vi "Non Linear Decimation on X by Min-Max Algorythm.vi"(6 "Width":u32, 8 "error in (no error)":errorcluster, 9 "Min Index":i32, 10 "Max Index":i32, 11 "Data To Decimate":dbl[](array[numeric])) -> (0 "error out":errorcluster, 3 "Decimated Data":dbl[](array[numeric]), 4 "Packet size":i32[](array[numeric]))   [LabVIEW 2022 SP3, in "Decimation.lvlib"]
uses:
  Decimation.lvlib
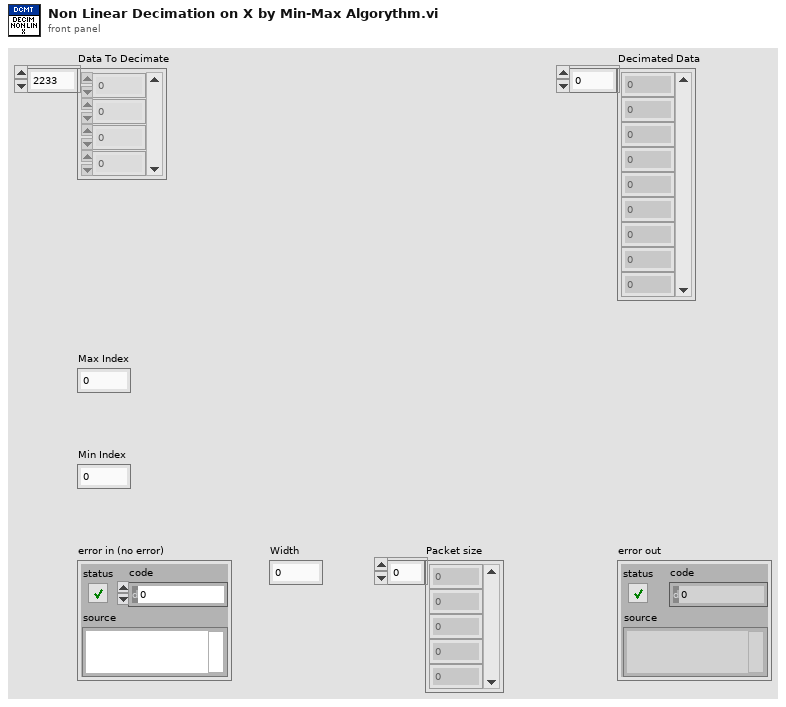
[diagram p1: front panel]
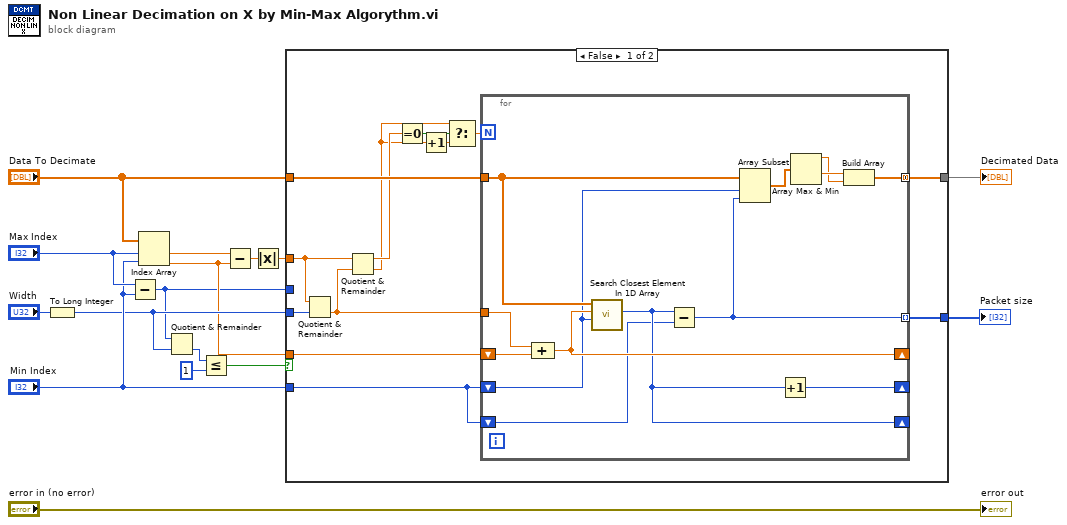
[diagram p0: block diagram]
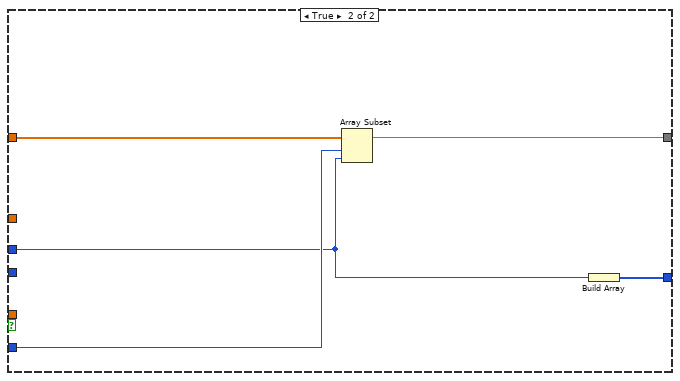
[diagram p2: hidden frame]
diagram:
  n1 = To Long Integer(number="Width") -> (32bit integer=w3:i32)
  n2 = Subtract(x="Max Index", y="Min Index") -> (x-y=w1:i32)
  n3 = Index Array(array="Data To Decimate", index #1="Max Index", index #2="Min Index") -> (element #1=w10:dbl, element #2=w2:dbl)
  n4 = Quotient & Remainder(x=w1, y=w3) -> (floor(x/y)=w6:i32)  [unwired: 1 out]
  n5 = Less Or Equal?(x=w6, y=1) -> (x <= y?=w12:bool)
  n6 = Subtract(x=w10, y=w2) -> (x-y=w11:dbl)
  n7 = Absolute Value(x=w11) -> (abs(x)=w7:dbl)
  n8 = case shown="False" w12 {
    tunnel: [w29 w46] -> w15
    tunnel: [w28 w44] -> w8
    tunnel: "Data To Decimate" -> [w25 w47]
    tunnel: w7 -> [w21 _]
    tunnel: "Min Index" -> [w17 w45]
    tunnel: w3 -> [w20 _]
    tunnel: w2 -> [w18 _]
    tunnel: w1 -> [_ w43]
    frame False {
      n9 = Quotient & Remainder(x=w21, y=w20) -> (floor(x/y)=w19:dbl)  [unwired: 1 out]
      n10 = Quotient & Remainder(x=w21, y=w19) -> (x-y*floor(x/y)=w24:dbl, floor(x/y)=w23:dbl)
      n11 = Equal To 0?(x=w24) -> (x = 0?=w27:bool)
      n12 = Increment(x=w23) -> (x+1=w26:dbl)
      n13 = Select(t=w23, s=w27, f=w26) -> (s? t:f=w22:dbl)
      n14 = for {
        N: w22 -> [_]
        tunnel: w19 -> [w36]
        tunnel: [w41] -> w29 mode=concatenating
        shift-right: [w39] -> _
        shift-left: w18 -> [w40]
        tunnel: [w30] -> w28 mode=indexing
        tunnel: w25 -> [w42]
        shift-right: [w34] -> _
        shift-left: w17 -> [w33]
        shift-right: [w32] -> _
        shift-left: w17 -> [w31]
        n15 = Compound Arithmetic op=ADD(w36, w40) -> (w39:dbl)
        n16 = call "Search Closest Element In 1D Array.vi"("Start index"=w33, "Desired element"=w39, "1D Array"=w42) -> ("Closest Index"=w32:i32)  [unwired: 7 in, 1 out]
        n17 = Subtract(x=w32, y=w31) -> (x-y=w30:i32)
        n18 = Array Subset(array=w42, index=w33, length=w30) -> (w35:dbl[])
        n19 = Increment(x=w32) -> (x+1=w34:i32)
        n20 = Array Max & Min(array=w35) -> (max value=w37:dbl, min value=w38:dbl)  [unwired: 2 out]
        n21 = Build Array(w38, w37) -> (w41:dbl[])
      }
    }
    frame True {
      n22 = Array Subset(array=w47, index=w45, length=w43) -> (w46:dbl[])
      n23 = Build Array(w43) -> (w44:i32[])
    }
  }
  "Decimated Data" <- w15
  "Packet size" <- w8
  "error out" <- "error in (no error)"
